vi "WriteTufts.vi"(1 "Text":T1={"Text"="Tufts", "Color Box"=12116735, "Alpha"=0.6, path "/Kim/Library/Fonts/Tahoma.ttf"}) -> (0 "Scene.Object Out":refnum<vi>)   [LabVIEW 2010]
uses:
  <vilib>/picture/3D Picture Control/NI_3D Picture Control.lvlib
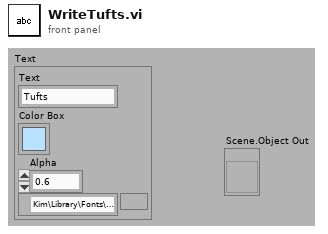
[diagram p1: front panel]
types:
  T1 = cluster{"Text":string, "Color Box":u32, "Alpha":sgl, path}
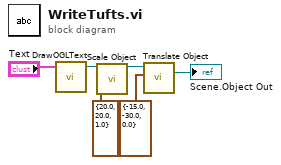
[diagram p0: block diagram]
diagram:
  n1 = call <userlib>:"DrawOGLText.vi"("Text"="Text") -> ("object out"=w5:refnum<vi>)  [unwired: 5 in, 1 out]
  n2 = call <vilib>:"Scale Object.vi"("Scale"=cluster{"X":sgl, "Y":sgl, "Z":sgl} {"X"=20.0, "Y"=20.0, "Z"=1.0}, "Scene.Object In"=w5) -> ("Scene.Object Out"=w2:refnum<vi>)  [unwired: 8 in, 1 out]
  n3 = call <vilib>:"Translate Object.vi"("Translation"=cluster{"X":sgl, "Y":sgl, "Z":sgl} {"X"=-15.0, "Y"=-30.0, "Z"=0.0}, "Scene.Object In"=w2) -> ("Scene.Object Out"=→"Scene.Object Out":refnum<vi>)  [unwired: 8 in, 1 out]
